vi "GetProtocolSection.vi"(8 "error in (no error)":errorcluster caption="에러 입력(에러 없음)", 10 "SectionMap":T1, 11 "ABFFIO IN":refnum<class "ABFFIO.lvclass">) -> (0 "error out":errorcluster caption="에러 출력", 3 "ABFFIO OUT":refnum<class "ABFFIO.lvclass">)   [LabVIEW 2017, in "ABFFIO.lvclass"]
uses:
  ABFFIO.lvclass
  ABFFIO.lvclass/ABFFIO.ctl
panel:
  out "SecPerPoint":dbl
  out "Samplingrate":i32
  out "MumSamplesPerEpisode":u32
  out "OperationMode":u8
  out "DACRange":sgl
  out "ADCRange":sgl
  out "ADCSequenceInterval":sgl
  out "DACResolution":u32
  out "ADCResolution":u32
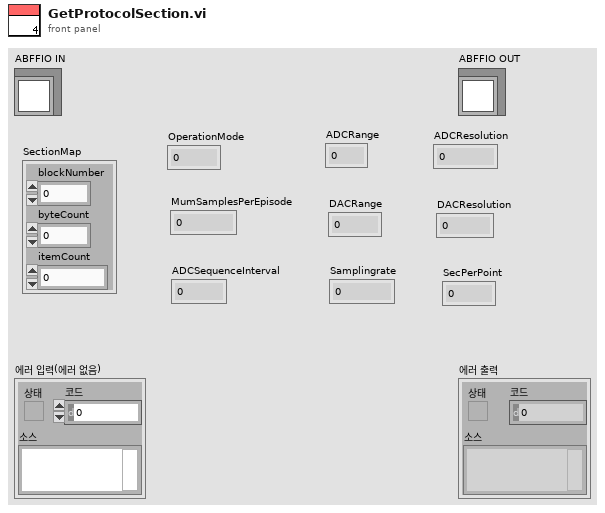
[diagram p1: front panel]
types:
  T1 = cluster{"blockNumber":u32, "byteCount":u32, "itemCount":u32}
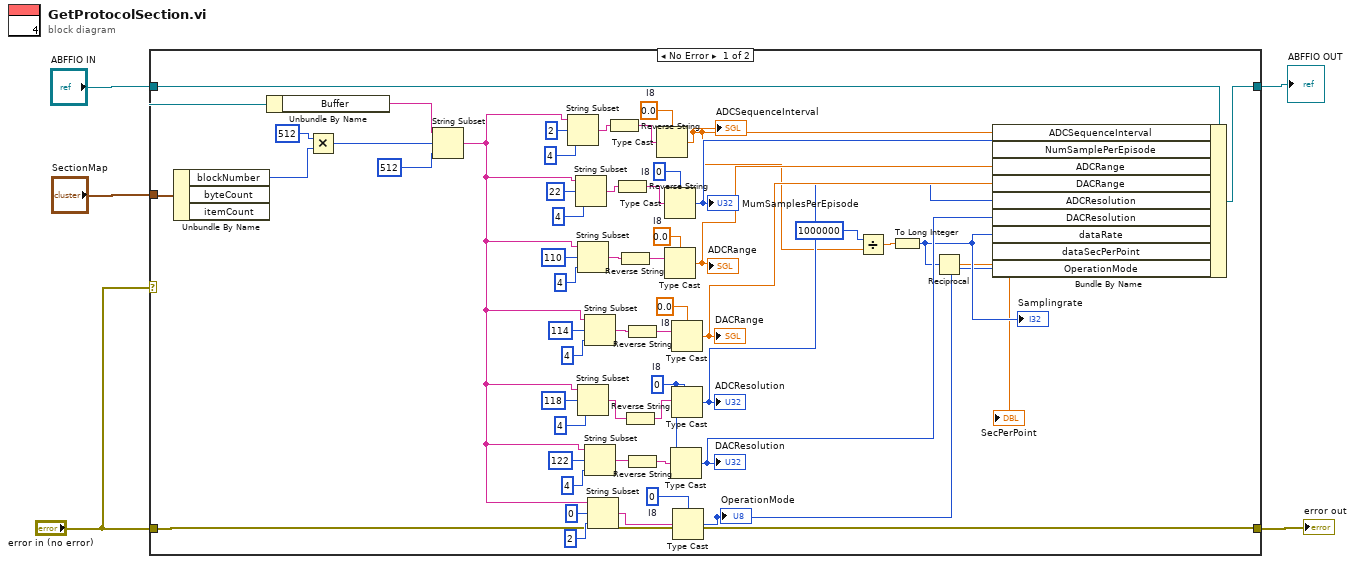
[diagram p0: block diagram]
diagram:
  n1 = case shown="No Error" "error in (no error)" {
    selector: "error in (no error)" -> [_ w61]
    tunnel: [w6 w61] -> w5
    tunnel: [w25 w60] -> w3
    tunnel: "ABFFIO IN" -> [w30 w60]
    tunnel: "SectionMap" -> [w36 _]
    tunnel: "error in (no error)" -> [w6 _]
    frame No Error {
      w19 = u32 0  # I8
      w21 = u8 0  # I8
      w31 = sgl 0.0  # I8
      w38 = sgl 0.0  # I8
      w39 = sgl 0.0  # I8
      w40 = u32 0  # I8
      n2 = Unbundle By Name(w36) -> ("blockNumber"=w59:u32)  [unwired: 2 out]
      n3 = Unbundle By Name(w30) -> ("Buffer"=w56:string)
      n4 = Multiply(x=512, y=w59) -> (x*y=w57:u32)
      n5 = String Subset(string=w56, offset (0)=w57, length (rest)=i16 512) -> (substring=w14:string)
      n6 = String Subset(string=w14, offset (0)=i16 2 ("오프셋(0)"), length (rest)=4 ("길이(나머지)")) -> (substring=w42:string)
      n7 = String Subset(string=w14, offset (0)=i16 22 ("오프셋(0)"), length (rest)=4 ("길이(나머지)")) -> (substring=w17:string)
      n8 = String Subset(string=w14, offset (0)=110 ("오프셋(0)"), length (rest)=4 ("길이(나머지)")) -> (substring=w48:string)
      n9 = String Subset(string=w14, offset (0)=i16 118 ("오프셋(0)"), length (rest)=4 ("길이(나머지)")) -> (substring=w53:string)
      n10 = String Subset(string=w14, offset (0)=114 ("오프셋(0)"), length (rest)=4 ("길이(나머지)")) -> (substring=w32:string)
      n11 = String Subset(string=w14, offset (0)=i16 122 ("오프셋(0)"), length (rest)=4 ("길이(나머지)")) -> (substring=w22:string)
      n12 = String Subset(string=w14, offset (0)=i16 0 ("오프셋(0)"), length (rest)=2 ("길이(나머지)")) -> (substring=w20:string)
      n13 = Reverse String(1:w42) -> (0:w41:string)
      n14 = Reverse String(1:w17) -> (0:w18:string)
      n15 = Reverse String(1:w48) -> (0:w37:string)
      n16 = Reverse String(1:w53) -> (0:w52:string)
      n17 = Reverse String(1:w32) -> (0:w35:string)
      n18 = Reverse String(1:w22) -> (0:w43:string)
      n19 = Type Cast(type=w39, x=w41) -> (*(type *) &x=w11:sgl)
      "ADCSequenceInterval" <- w11
      n20 = Type Cast(type=w19, x=w18) -> (*(type *) &x=w13:u32)
      "MumSamplesPerEpisode" <- w13
      n21 = Type Cast(type=w38, x=w37) -> (*(type *) &x=w29:sgl)
      "ADCRange" <- w29
      n22 = Type Cast(type=w40, x=w43) -> (*(type *) &x=w26:u32)
      "DACResolution" <- w26
      n23 = Type Cast(type=w31, x=w35) -> (*(type *) &x=w28:sgl)
      "DACRange" <- w28
      n24 = Type Cast(type=w40, x=w52) -> (*(type *) &x=w27:u32)
      "ADCResolution" <- w27
      n25 = Type Cast(type=w21, x=w20) -> (*(type *) &x=w7:u8)
      "OperationMode" <- w7
      n26 = Divide(x=1000000, y=w11) -> (x/y=w10:sgl)
      n27 = To Long Integer(number=w10) -> (32bit integer=w9:i32)
      "Samplingrate" <- w9
      n28 = Reciprocal(x=w9) -> (1/x=w8:dbl)
      "SecPerPoint" <- w8
      n29 = Bundle By Name(cluster=w30, "ADCSequenceInterval"=w11, "NumSamplePerEpisode"=w13, "ADCRange"=w29, "DACRange"=w28, "ADCResolution"=w27, "DACResolution"=w26, "dataRate"=w9, "dataSecPerPoint"=w8, "OperationMode"=w7) -> (w25:refnum<class "ABFFIO.lvclass">)
    }
    frame Error {
    }
  }
  "error out" <- w5
  "ABFFIO OUT" <- w3
